vi "test_objectArray.vi"(8 "error in (no error)":errorcluster) -> (0 "error out":errorcluster)   [LabVIEW 2013]
uses:
  test-TestableClass/Caraya-TestableClass.lvclass
  test-TestableClass/Caraya-TestableClass.lvclass/Caraya-TestableClass.ctl
  <vilib>/Utility/sysdir.llb/System Directory Type.ctl
  Run Test (Object Array).vi
  Caraya.lvlib
panel:
  in  "Report Type":enum16{"None", "Default (txt)", "JUnit (xml)"}(ring)
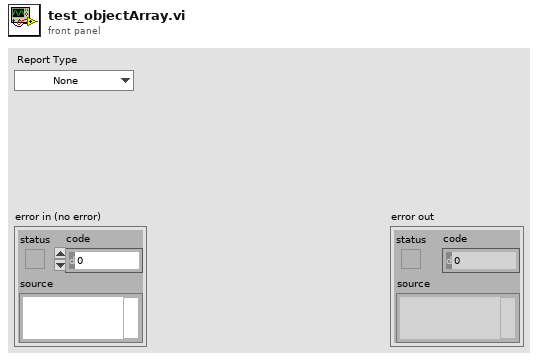
[diagram p1: front panel]
types:
  T1 = typedef "System Directory Type.ctl" = i32
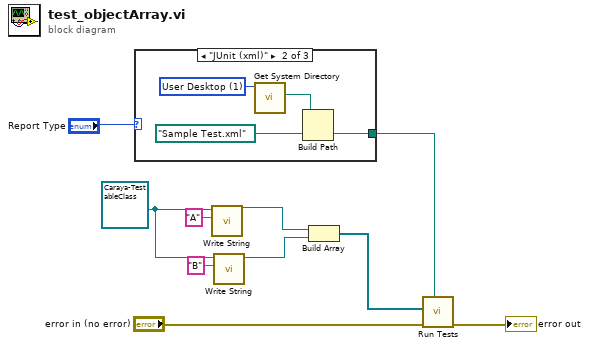
[diagram p0: block diagram]
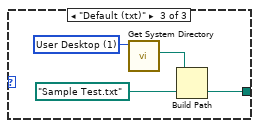
[diagram p3: hidden frame]
diagram:
  w7 = refnum<class "Caraya-TestableClass.lvclass"> refnum ("Caraya-TestableClass.lvclass")
  n1 = case shown="\"JUnit (xml)\"" "Report Type" {
    tunnel: [_ w11 w15] -> w1
    frame "None", Default {
    }
    frame "JUnit (xml)" {
      w13 = T1 1 items=["User Home"=0, "User Desktop"=1, "User Documents"=2, "User Application Data"=3, "User Preferences"=4, "User Temporary"=5, "Public Documents"=6, "Public Application Data"=7, "Public Preferences"=8, "Public Cache"=13, "System Core Libraries"=9, "System Installed Libraries"=10, "Application Files"=11, "Boot Volume Root"=12] ("system directory type")
      n2 = call <vilib>:"Get System Directory.vi"("system directory type"=w13) -> ("system directory"=w12:path)  [unwired: 10 in]
      n3 = Build Path(base path=w12, name or relative path=path "Sample Test.xml" ("Report Path")) -> (appended path=w11:path)
    }
    frame "Default (txt)" {
      w17 = T1 1 items=["User Home"=0, "User Desktop"=1, "User Documents"=2, "User Application Data"=3, "User Preferences"=4, "User Temporary"=5, "Public Documents"=6, "Public Application Data"=7, "Public Preferences"=8, "Public Cache"=13, "System Core Libraries"=9, "System Installed Libraries"=10, "Application Files"=11, "Boot Volume Root"=12] ("system directory type")
      n4 = call <vilib>:"Get System Directory.vi"("system directory type"=w17) -> ("system directory"=w16:path)  [unwired: 10 in]
      n5 = Build Path(base path=w16, name or relative path=path "Sample Test.txt" ("Report Path")) -> (appended path=w15:path)
    }
  }
  n6 = call "Write String.vi"("String"="A", "Caraya-TestableClass in"=w7) -> ("Caraya-TestableClass out"=w4:refnum<class "Caraya-TestableClass.lvclass">)  [unwired: 9 in]
  n7 = call "Write String.vi"("String"="B", "Caraya-TestableClass in"=w7) -> ("Caraya-TestableClass out"=w3:refnum<class "Caraya-TestableClass.lvclass">)  [unwired: 9 in]
  n8 = Build Array(w4, w3) -> (w8:refnum<class "Caraya-TestableClass.lvclass">[])
  n9 = call-poly "Run Tests.vi"("Report Path"=w1, "error in"="error in (no error)", "Objects"=w8) -> ("error out"=→"error out":errorcluster)  [unwired: 8 in]
